vi "Spartan HTTP Load Default Document.vi"(7 "url path":string, 8 "error in (no error)":errorcluster, 9 "script alias":bool, 10 "absolut path":string, 11 "HTTP Data":T1 {"object data"."time" format="%0.2f"}) -> (0 "error out":errorcluster, 3 "Reply":T4)   [LabVIEW 2011]
uses:
  ITK EXT/http/cgi.llb/CGI Reply.ctl
  Spartan HTTP Session.ctl
  ITK EXT/http/http_obj.llb/HTTP Session Data.ctl
  ITK EXT/utils/keyedarr.llb/Keyed Array.ctl
  ITK EXT/http/config.llb/HTTP SRM.vi
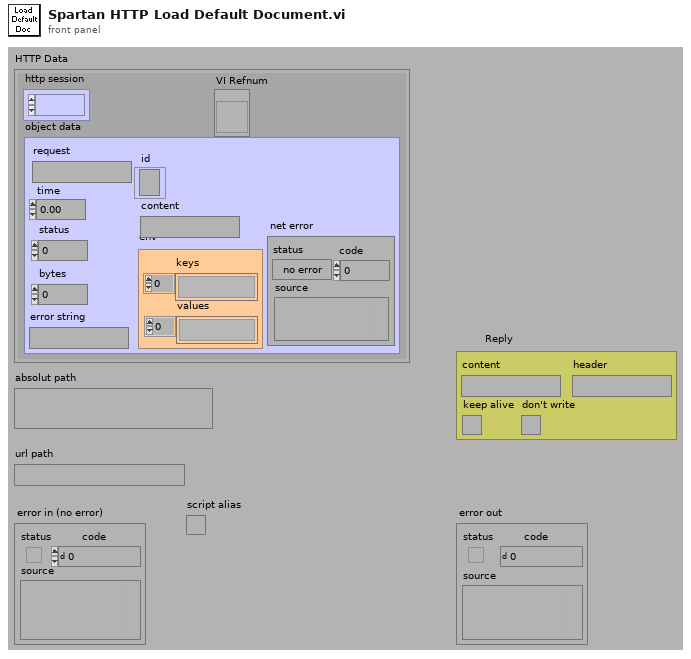
[diagram p1: front panel]
types:
  T1 = typedef "Spartan HTTP Session.ctl" = cluster{"http session":refnum<k1>, "object data":T2, "VI Refnum":refnum<vi>}
  T2 = typedef "HTTP Session Data.ctl" = cluster{"request":string, "time":dbl, "status":i32, "error string":string, "bytes":i32, "env":T3, "content":string, "id":refnum<k5>, "net error":errorcluster}
  T3 = typedef "Keyed Array.ctl" = cluster{"keys":string[], "values":string[]}
  T4 = typedef "CGI Reply.ctl" = cluster{"content":string, "header":string, "keep alive":bool, "don't write":bool}
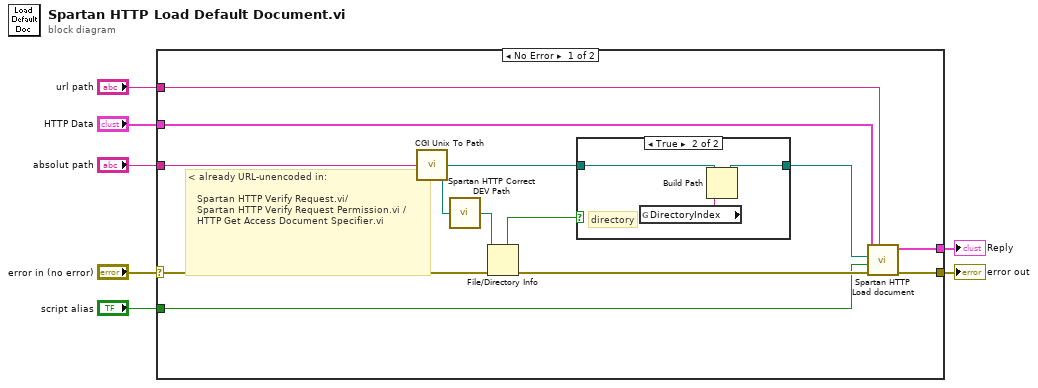
[diagram p0: block diagram]
diagram:
  n1 = case shown="No Error" "error in (no error)" {
    selector: "error in (no error)" -> [w17 w24]
    tunnel: [w19 _] -> w7
    tunnel: [w18 w24] -> w5
    tunnel: "absolut path" -> [w8 _]
    tunnel: "HTTP Data" -> [w15 _]
    tunnel: "url path" -> [w14 _]
    tunnel: "script alias" -> [w13 _]
    frame No Error {
      # "< already URL-unencoded in:\n\n   Spartan HTTP Verify Request.vi/\n   Spartan HTTP Verify Request Permission.vi /\n   HTTP Get Access Document Specifier.vi"
      n2 = call "CGI Unix To Path.vi"("unix path"=w8) -> ("platform path"=w11:path)  [unwired: 1 out]
      n3 = call "Spartan HTTP Correct DEV Path.vi"("Normal Path"=w11) -> ("Dev Corrected Path"=w12:path)  [unwired: 4 out]
      n4 = File/Directory Info(path=w12, error in=w17) -> (directory=w10:bool, error out=w16:errorcluster)  [unwired: 5 out]
      n5 = case shown="True" w10 {
        tunnel: w11 -> [w20 w23]
        tunnel: [w20 w21] -> w9
        frame False {
          # "it's a file"
        }
        frame True {
          # "directory"
          n6 = global read "HTTP SRM.vi" "DirectoryIndex"() -> (w22:string)
          n7 = Build Path(base path=w23, name or relative path=w22) -> (appended path=w21:path)
        }
      }
      n8 = call "Spartan HTTP Load document.vi"("url path"=w14, "error in (no error)"=w16, "script alias"=w13, "File Path"=w9, "HTTP Data"=w15) -> ("error out"=w18:errorcluster, "Reply"=w19:T4)  [unwired: 5 out]
    }
    frame Error {
    }
  }
  "Reply" <- w7
  "error out" <- w5
